vi "Make DLL Param(Read Profile Rsp).vi"(1 "Read Profile Rsp 2":T1) -> (0 "pRsp":T2)   [LabVIEW 2015, in "KEYENCE LJ-X8000A.lvlib"]
uses:
  KEYENCE LJ-X8000A.lvlib
  Public/Clusters/Read Profile Rsp.ctl
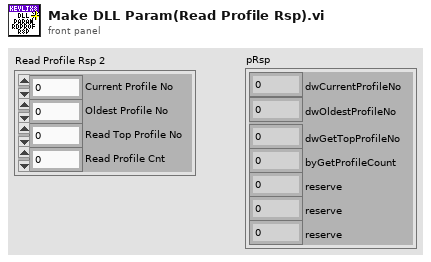
[diagram p1: front panel]
types:
  T1 = typedef "KEYENCE LJ-X8000A.lvlib/Read Profile Rsp.ctl" = cluster{"Current Profile No":u32, "Oldest Profile No":u32, "Read Top Profile No":u32, "Read Profile Cnt":u8}
  T2 = cluster{"dwCurrentProfileNo":u32, "dwOldestProfileNo":u32, "dwGetTopProfileNo":u32, "byGetProfileCount":u8, "reserve":u8, "reserve":u8, "reserve":u8}
  T3 = cluster{"Current Profile No":u32, "Oldest Profile No":u32, "Read Top Profile No":u32, "Read Profile Cnt":u8, "reserve":u8, "reserve":u8, "reserve":u8}
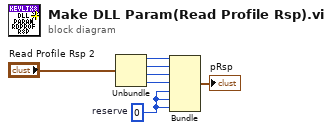
[diagram p0: block diagram]
diagram:
  w3 = u8 0  # reserve
  n1 = Unbundle("Read Profile Rsp 2") -> ("Current Profile No"=w7:u32, "Oldest Profile No"=w6:u32, "Read Top Profile No"=w5:u32, "Read Profile Cnt"=w4:u8)
  n2 = Bundle("Current Profile No"=w7, "Oldest Profile No"=w6, "Read Top Profile No"=w5, "Read Profile Cnt"=w4, "reserve"=w3, "reserve"=w3, "reserve"=w3) -> (→"pRsp":T3)  [unwired: 1 in]
